vi "test-numerical-jacobian.vi"(8 "error in (no error)":errorcluster) -> (0 "error out":errorcluster, 3 "ALL Tests Passed":bool)   [LabVIEW 2019]
uses:
  <vilib>/Analysis/Matrix/Datatypes/RealMatrix.ctl
  <vilib>/Rock Robotics/WPI/ThirdParty/JAS_Junk/TrajLib/MatBuilder_Create.vi
  <vilib>/Rock Robotics/WPI/ThirdParty/JAS_Junk/TrajLib/Trajectory_Library.lvlib
  <vilib>/Analysis/Matrix/NI_Matrix.lvlib
panel:
  out "TEst Passed 0":bool
  out "TEst Passed 1":bool
  out "D":T1
  out "Error 1":bool
  out "Result 1":T1
  out "A":T1
  out "Error 0":bool
  out "Result 0":T1
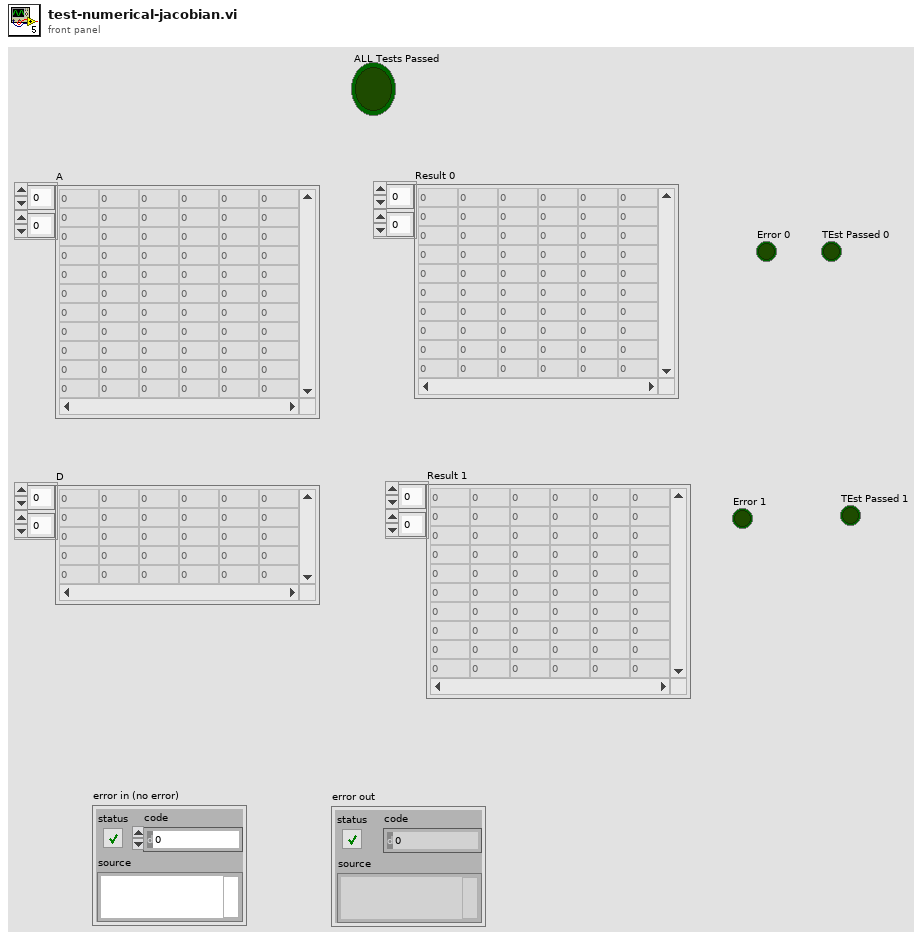
[diagram p1: front panel]
types:
  T1 = typedef "NI_Matrix.lvlib/RealMatrix.ctl" = dbl[][]
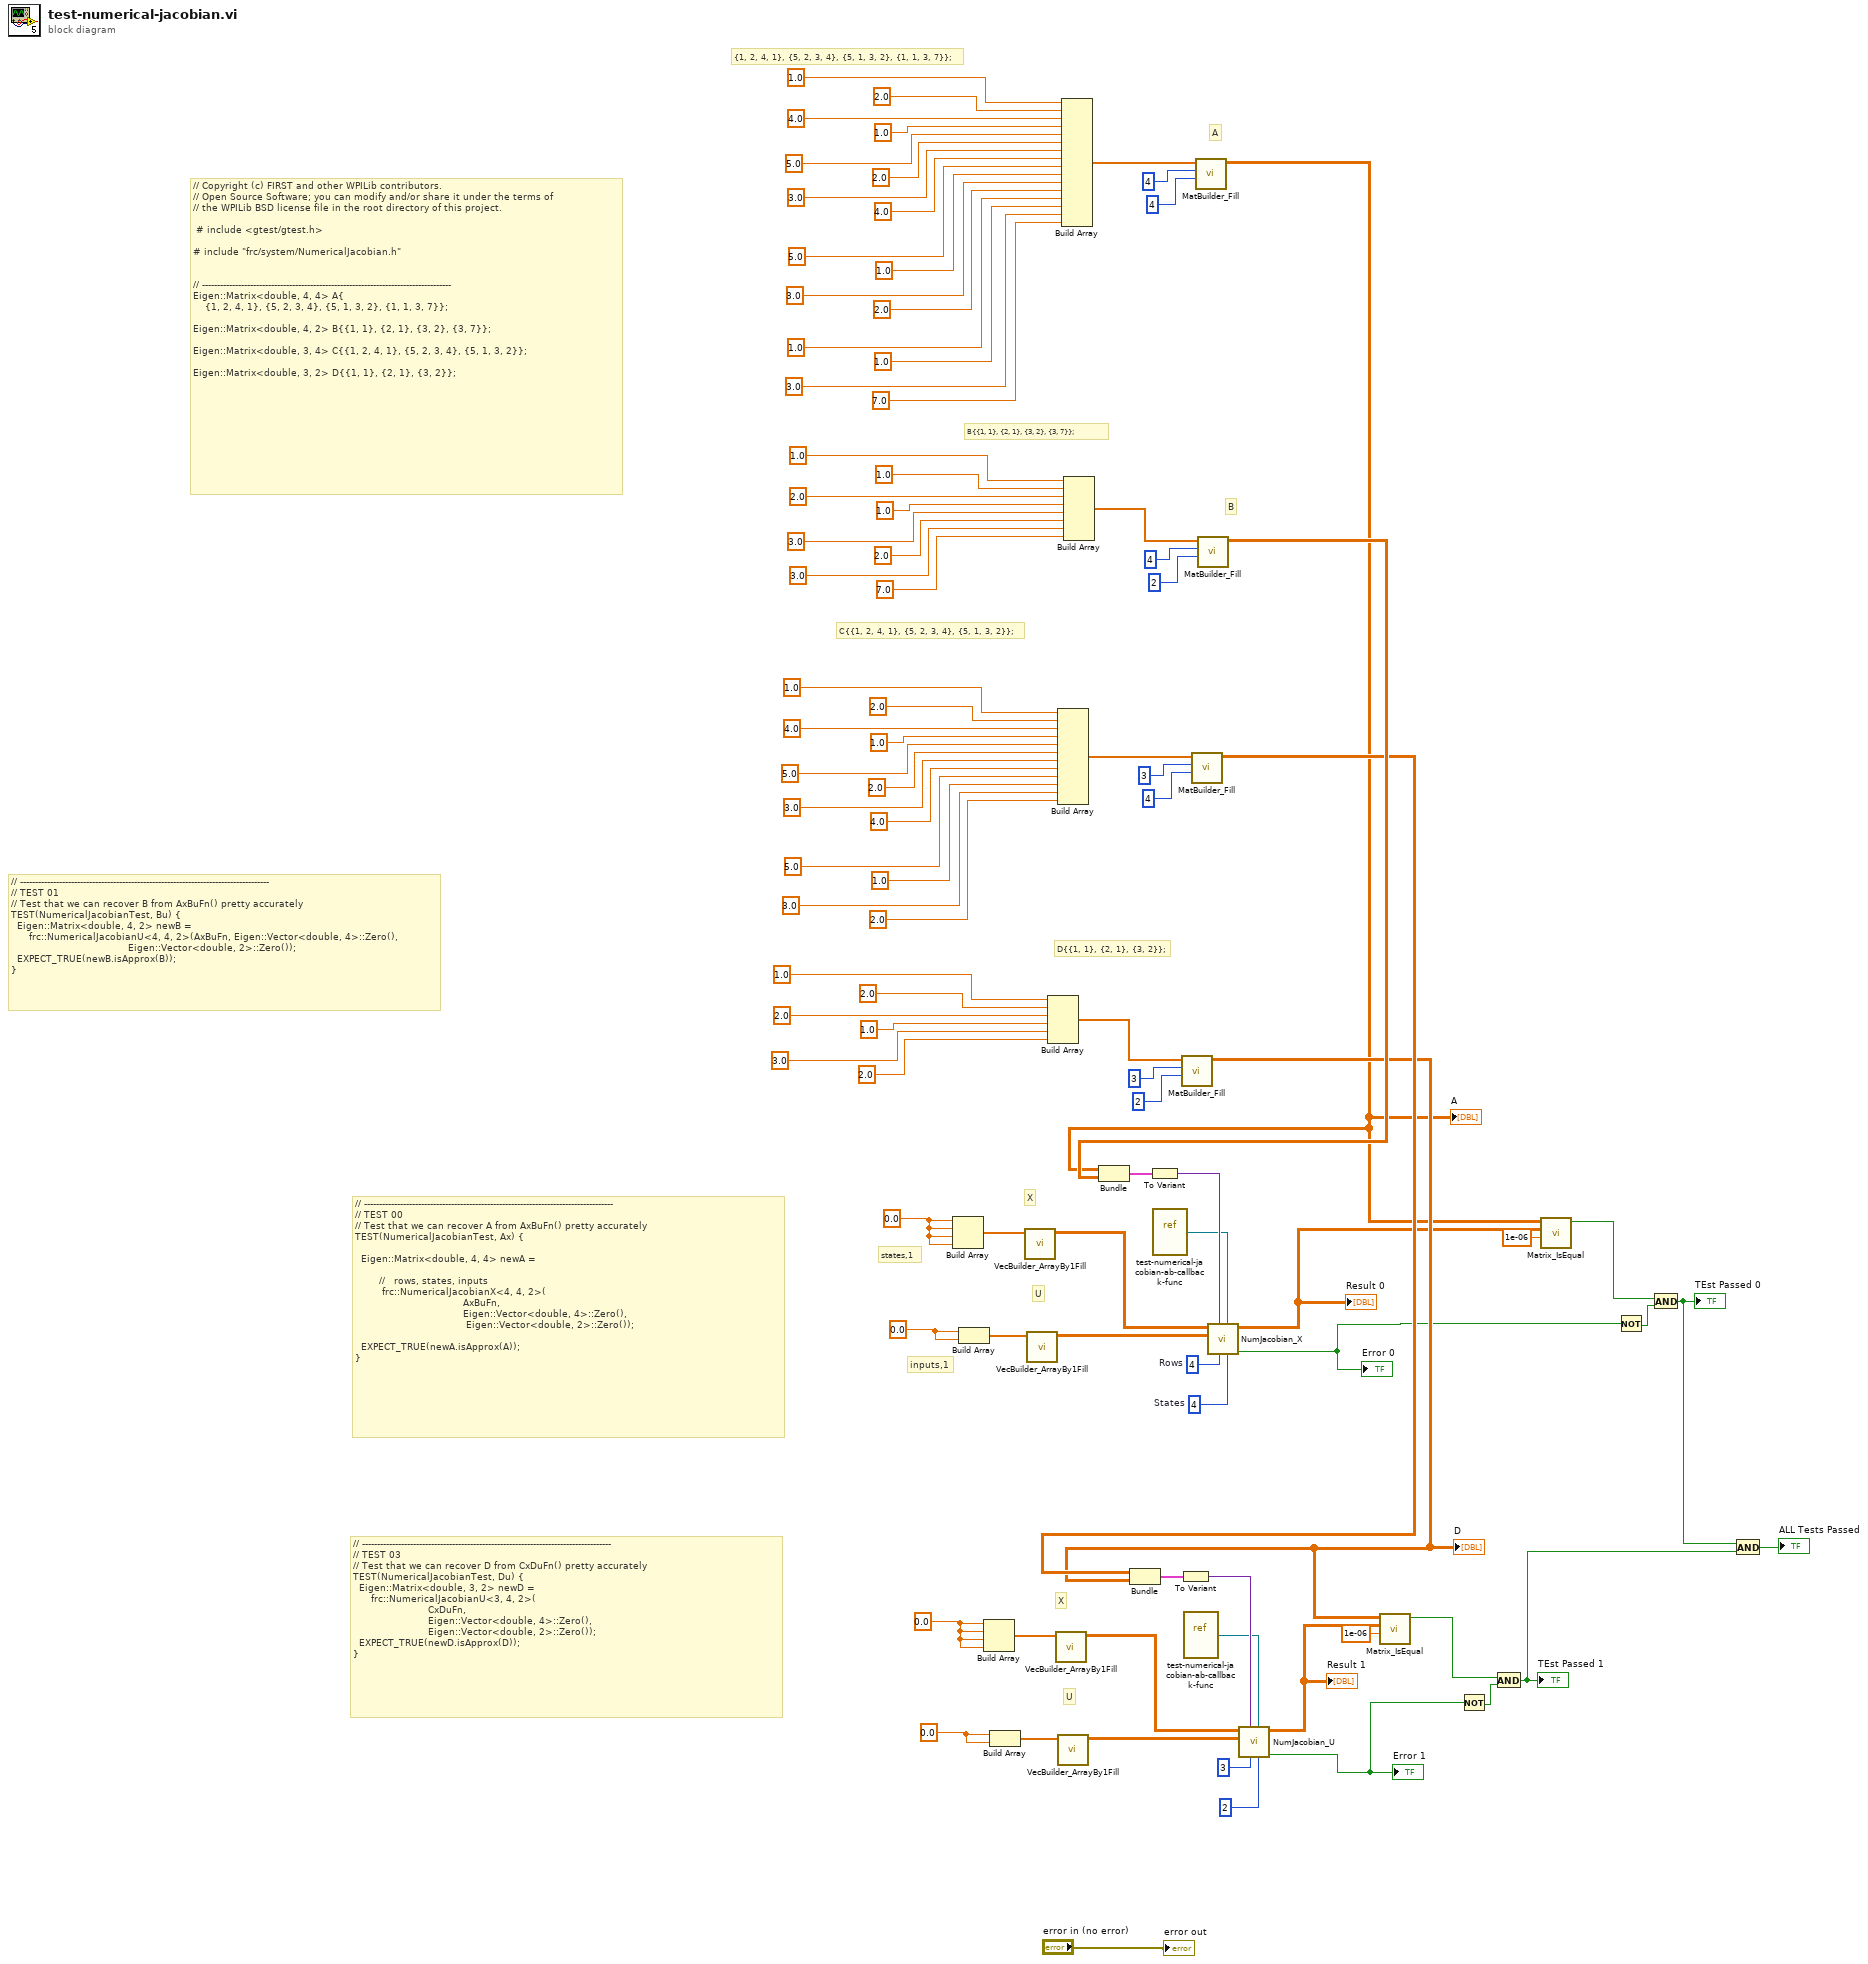
[diagram p0: block diagram]
diagram:
  w25 = 0.0 ("element")
  w27 = 0.0 ("element")
  w29 = 4  # States
  w30 = 4  # Rows
  w37 = 0.0 ("element")
  w39 = 0.0 ("element")
  # "inputs,1"
  # "states,1"
  # "U"
  # "X"
  # "B"
  # "A"
  # "U"
  # "X"
  # "D{{1, 1}, {2, 1}, {3, 2}};"
  # "C{{1, 2, 4, 1}, {5, 2, 3, 4}, {5, 1, 3, 2}};"
  # "B{{1, 1}, {2, 1}, {3, 2}, {3, 7}};"
  # "{1, 2, 4, 1}, {5, 2, 3, 4}, {5, 1, 3, 2}, {1, 1, 3, 7}};"
  # "// -----------------------------------------------------------------------------------\n// TEST 00\n// Test that we can recover A from AxBuFn() pretty accurately\nTEST(NumericalJacobianTest, Ax) {\n\n  Eigen::Matrix<double, 4, 4> newA =\n     \n        //   rows, states, inputs \n         frc::NumericalJacobianX<4, 4, 2>(\n                                    AxBuFn, \n                                    Eigen::Vector<double, 4>::Zero(),\n                                     Eigen::Vector<double, 2>::Zero());\n\n  EXPECT_TRUE(newA.isApprox(A));\n}"
  # "// -----------------------------------------------------------------------------------\n// TEST 01\n// Test that we can recover B from AxBuFn() pretty accurately\nTEST(NumericalJacobianTest, Bu) {\n  Eigen::Matrix<double, 4, 2> newB =\n      frc::NumericalJacobianU<4, 4, 2>(AxBuFn, Eigen::Vector<double, 4>::Zero(),\n                                       Eigen::Vector<double, 2>::Zero());\n  EXPECT_TRUE(newB.isApprox(B));\n}"
  # "// -----------------------------------------------------------------------------------\n// TEST 03\n// Test that we can recover D from CxDuFn() pretty accurately\nTEST(NumericalJacobianTest, Du) {\n  Eigen::Matrix<double, 3, 2> newD =\n      frc::NumericalJacobianU<3, 4, 2>(\n                         CxDuFn, \n                         Eigen::Vector<double, 4>::Zero(),\n                         Eigen::Vector<double, 2>::Zero());\n  EXPECT_TRUE(newD.isApprox(D));\n}"
  # "// Copyright (c) FIRST and other WPILib contributors.\n// Open Source Software; you can modify and/or share it under the terms of\n// the WPILib BSD license file in the root directory of this project.\n\n # include <gtest/gtest.h>\n\n# include \"frc/system/NumericalJacobian.h\"\n\n\n// -----------------------------------------------------------------------------------\nEigen::Matrix<double, 4, 4> A{\n    {1, 2, 4, 1}, {5, 2, 3, 4}, {5, 1, 3, 2}, {1, 1, 3, 7}};\n\nEigen::Matrix<double, 4, 2> B{{1, 1}, {2, 1}, {3, 2}, {3, 7}};\n\nEigen::Matrix<double, 3, 4> C{{1, 2, 4, 1}, {5, 2, 3, 4}, {5, 1, 3, 2}};\n\nEigen::Matrix<double, 3, 2> D{{1, 1}, {2, 1}, {3, 2}};"
  n1 = Build Array(w39, w39, w39, w39) -> (w40:dbl[])
  n2 = Build Array(w37, w37) -> (w38:dbl[])
  n3 = Build Array(w27, w27, w27, w27) -> (w28:dbl[])
  n4 = Build Array(w25, w25) -> (w26:dbl[])
  n5 = call <vilib>:"VecBuilder_ArrayBy1Fill.vi"("R Array"=w40) -> ("Output Vector"=w36:T1)  [unwired: 10 in]
  n6 = call <vilib>:"VecBuilder_ArrayBy1Fill.vi"("R Array"=w38) -> ("Output Vector"=w35:T1)  [unwired: 10 in]
  n7 = Build Array(1.0 ("element"), 2.0 ("element"), 2.0 ("element"), 1.0 ("element"), 3.0 ("element"), 2.0 ("element")) -> (w49:dbl[])
  n8 = call <vilib>:"VecBuilder_ArrayBy1Fill.vi"("R Array"=w28) -> ("Output Vector"=w24:T1)  [unwired: 10 in]
  n9 = Build Array(1.0 ("element"), 2.0 ("element"), 4.0 ("element"), 1.0 ("element"), 5.0 ("element"), 2.0 ("element"), 3.0 ("element"), 4.0 ("element"), 5.0 ("element"), 1.0 ("element"), 3.0 ("element"), 2.0 ("element")) -> (w64:dbl[])
  n10 = call <vilib>:"VecBuilder_ArrayBy1Fill.vi"("R Array"=w26) -> ("Output Vector"=w23:T1)  [unwired: 10 in]
  n11 = Build Array(1.0 ("element"), 2.0 ("element"), 4.0 ("element"), 1.0 ("element"), 5.0 ("element"), 2.0 ("element"), 3.0 ("element"), 4.0 ("element"), 5.0 ("element"), 1.0 ("element"), 3.0 ("element"), 2.0 ("element"), 1.0 ("element"), 1.0 ("element"), 3.0 ("element"), 7.0 ("element")) -> (w94:dbl[])
  n12 = Build Array(1.0 ("element"), 1.0 ("element"), 2.0 ("element"), 1.0 ("element"), 3.0 ("element"), 2.0 ("element"), 3.0 ("element"), 7.0 ("element")) -> (w75:dbl[])
  n13 = vi-ref "test-numerical-jacobian-ab-callback-func.vi"() -> (w31:refnum<vi>)
  n14 = call <vilib>:"MatBuilder_Fill.vi"("Columns"=2, "Rows"=3, "Value List"=w49) -> ("output matrix"=w16:T1)  [unwired: 8 in]
  "D" <- w16
  n15 = vi-ref "test-numerical-jacobian-ab-callback-func.vi"() -> (w20:refnum<vi>)
  n16 = call <vilib>:"MatBuilder_Fill.vi"("Columns"=4, "Rows"=3, "Value List"=w64) -> ("output matrix"=w17:T1)  [unwired: 8 in]
  n17 = Bundle("output matrix"=w17, "output matrix"=w16) -> (w22:cluster{"output matrix":T1, "output matrix":T1})  [unwired: 1 in]
  n18 = To Variant(anything=w22) -> (Variant=w21:variant)
  n19 = call <vilib>:"MatBuilder_Fill.vi"("Columns"=4, "Rows"=4, "Value List"=w94) -> ("output matrix"=w7:T1)  [unwired: 8 in]
  "A" <- w7
  n20 = call <vilib>:"MatBuilder_Fill.vi"("Columns"=2, "Rows"=4, "Value List"=w75) -> ("output matrix"=w34:T1)  [unwired: 8 in]
  n21 = Bundle("output matrix"=w7, "output matrix"=w34) -> (w33:cluster{"output matrix":T1, "output matrix":T1})  [unwired: 1 in]
  n22 = To Variant(anything=w33) -> (Variant=w32:variant)
  n23 = call <vilib>:"NumJacobian_X.vi"("States"=w29, "F_FUNC"=w31, "Rows"=w30, "ExtraPassedData"=w32, "U"=w35, "X"=w36) -> ("Error"=w5:bool, "Result"=w6:T1)  [unwired: 4 in]
  "Result 0" <- w6
  "Error 0" <- w5
  n24 = call <vilib>:"NumJacobian_U.vi"("Inputs"=2 ("States"), "F_FUNC"=w20, "Rows"=3, "ExtraPassedData"=w21, "U"=w23, "X"=w24) -> ("Error"=w12:bool, "Result"=w15:T1)  [unwired: 4 in]
  "Result 1" <- w15
  "Error 1" <- w12
  n25 = call <vilib>:"Matrix_IsEqual.vi"("Tolerance"=1e-06, "other"=w15, "input matrix"=w16) -> ("Equal"=w13:bool)  [unwired: 8 in]
  n26 = Not(x=w12) -> (.not. x?=w11:bool)
  n27 = And(x=w13, y=w11) -> (x .and. y?=w2:bool)
  "TEst Passed 1" <- w2
  n28 = call <vilib>:"Matrix_IsEqual.vi"("Tolerance"=1e-06, "other"=w6, "input matrix"=w7) -> ("Equal"=w9:bool)  [unwired: 8 in]
  n29 = Not(x=w5) -> (.not. x?=w8:bool)
  n30 = And(x=w9, y=w8) -> (x .and. y?=w3:bool)
  "TEst Passed 0" <- w3
  n31 = And(x=w3, y=w2) -> (x .and. y?=→"ALL Tests Passed":bool)
  "error out" <- "error in (no error)"
